vi "DI.vi"(8 "error in":errorcluster caption="错误输入", 10 "Line":string(combo)="port0/line0", 11 "Device":tag="Dev7") -> (0 "error out":errorcluster caption="错误输出", 3 "data":bool caption="result")   [LabVIEW 2013]
uses:
  <vilib>/DAQmx/read.llb/DAQmx Read (Digital Bool 1Line 1Point).vi
  <vilib>/DAQmx/create/channels.llb/DAQmx Create Channel (DI-Digital Input).vi
  <vilib>/DAQmx/miscellaneous.llb/DAQmx Fill In Error Info.vi
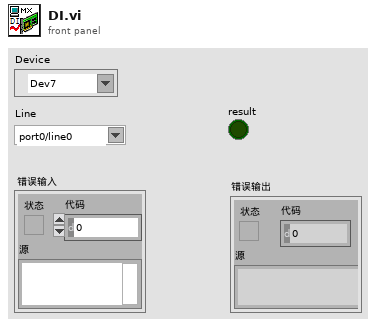
[diagram p1: front panel]
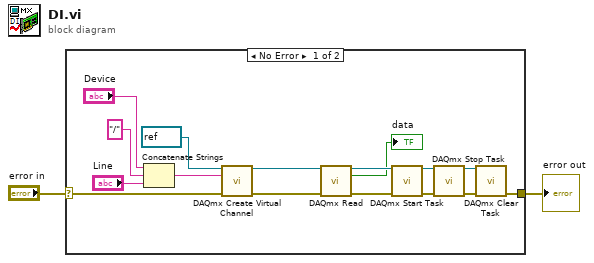
[diagram p0: block diagram]
diagram:
  n1 = case shown="No Error" "error in" {
    selector: "error in" -> [w3 w19]
    tunnel: [w9 w19] -> w2
    frame No Error {
      n2 = Concatenate Strings("Device", "/" ("字符串"), "Line") -> (w8:string)
      n3 = call-poly <vilib>:"DAQmx Create Virtual Channel.vi"("task in"=refnum<k21> refnum, "lines"=w8, "error in"=w3) -> ("task out"=w16:refnum<k21>, "error out"=w6:errorcluster)  [unwired: 11 in]
      n4 = call-poly <vilib>:"DAQmx Read.vi"("task/channels in"=w16, "error in"=w6) -> ("task out"=w14:refnum<k21>, "data"=→"data":bool, "error out"=w5:errorcluster)  [unwired: 11 in]
      n5 = call <vilib>:"DAQmx Start Task.vi"("task/channels in"=w14, "error in"=w5) -> ("task out"=w13:refnum<k21>, "error out"=w12:errorcluster)  [unwired: 12 in]
      n6 = call <vilib>:"DAQmx Stop Task.vi"("task/channels in"=w13, "error in"=w12) -> ("task out"=w11:refnum<k21>, "error out"=w10:errorcluster)  [unwired: 12 in]
      n7 = call <vilib>:"DAQmx Clear Task.vi"("task in"=w11, "error in"=w10) -> ("error out"=w9:errorcluster)  [unwired: 13 in]
    }
    frame Error {
    }
  }
  "error out" <- w2
